vi "CIE2T-Config.vi"(0 "AO Channels":i32[](array[numeric]), 1 "Attenuation (dB)":dbl[](array[numeric]), 5 "DP Freqs":T1, 7 "Sampling Rate (Hz)":dbl=100000.0, 9 "Duration (s)":dbl=0.1, 11 "error in (no error)":errorcluster, 12 "Ear":T2) -> (2 "dt (ms)":dbl, 3 "df (kHz)":dbl, 4 "coerced f1 (kHz)":dbl, 6 "coerced f2 (kHz)":dbl, 10 "Mic Avg":dbl[][](array[numeric]), 15 "error out":errorcluster)   [LabVIEW 2020]
uses:
  Utility VIs/Type Defs/Left-Right ring.ctl
  Cochlear Function Test Suite/LV Source/DPOAE VIs/Typedefs/DP-Freqs.ctl
  Misc VIs/Connection Manager/Type Defs/Input sources.ctl
  PXI DAQ VIs/DAQ Engine VIs/PXI Globals.vi
  PXI DAQ VIs/DAQ Engine VIs/AO Gain and Multiplier VIs/PXI Multipliers to AO Gains (1D).vi
  PXI DAQ VIs/TDT VIs/TDT-Signal Bank Action.ctl
  Utility VIs/Math VIs/dB to Linear (scalar).vi
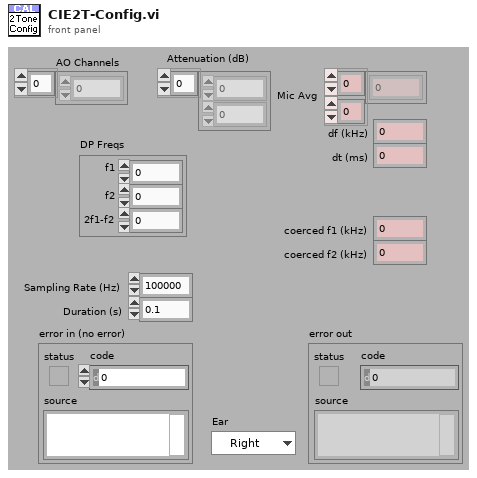
[diagram p1: front panel]
types:
  T1 = typedef "DP-Freqs.ctl" = cluster{"f1":dbl, "f2":dbl, "2f1-f2":dbl}
  T2 = typedef "Left-Right ring.ctl" = enum16{"Right", "Left"}
  T3 = typedef "Input sources.ctl" = u16
  T4 = typedef "TDT-Signal Bank Action.ctl" = enum16{"Init", "Write", "Read", "Rewrite", "Reset", "Recycle", "Ramp up", "Ramp down", "Zero"}
  T5 = typedef "TDT-Device Config.ctl" = cluster{"Output":T6, "Input":T8}
  T6 = typedef "TDT-Output source.ctl" = cluster{"Device":T7, "Num":i32}
  T7 = typedef "TDT-Device ID.ctl" = enum16{"None", "PA5", "RP2", "RL2", "RA16", "RV8", "RX5", "RX6", "RX7", "RX8", "RZ2", "RZ5", "RZ6"}
  T8 = typedef "TDT-Input source.ctl" = enum16{"Front Panel", "RA4LI", "RA16LI"}
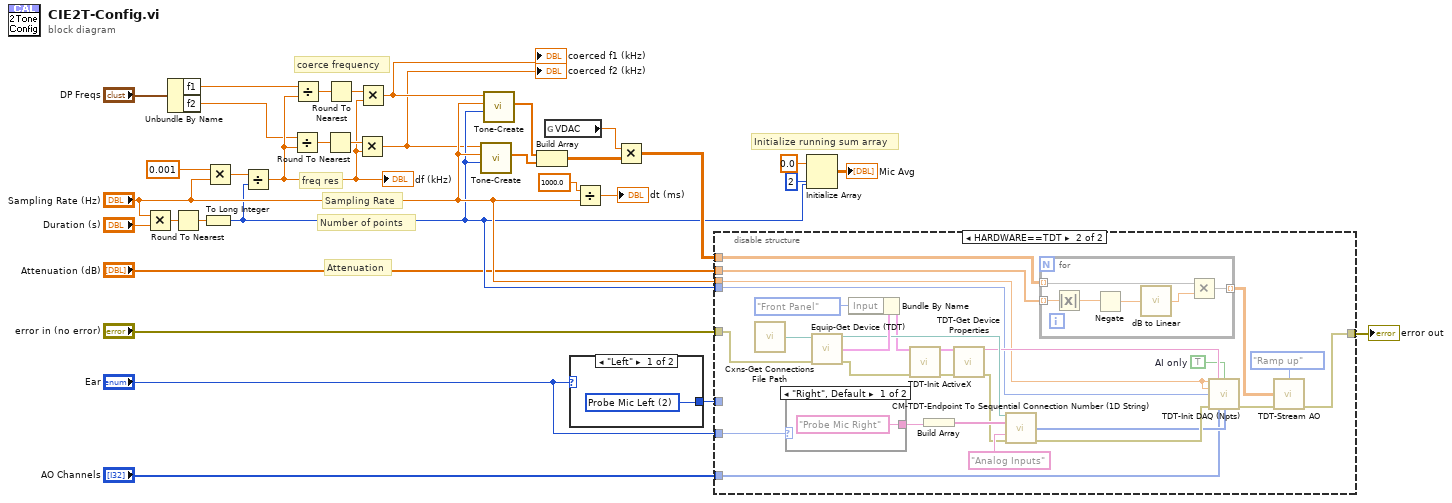
[diagram p0: block diagram]
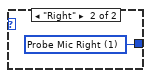
[diagram p2: hidden frame]
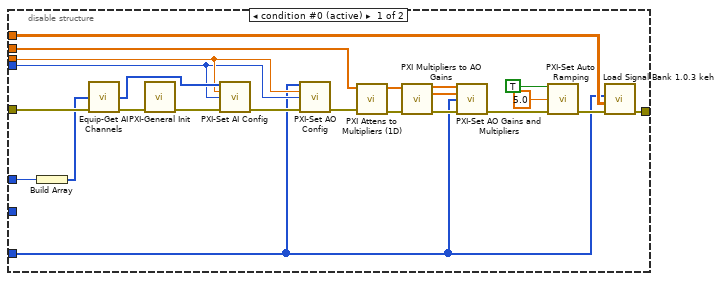
[diagram p3: hidden frame]
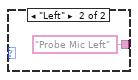
[diagram p4: hidden frame]
diagram:
  # "freq res"
  # "Attenuation"
  # "Sampling Rate"
  # "coerce frequency"
  # "Number of points"
  # "Initialize running sum array"
  n1 = Multiply(x="Sampling Rate (Hz)", y="Duration (s)") -> (x*y=w27:dbl)
  n2 = Unbundle By Name("DP Freqs") -> ("f1"=w6:dbl, "f2"=w5:dbl)
  n3 = Round To Nearest(number=w27) -> (nearest integer value=w26:dbl)
  n4 = To Long Integer(number=w26) -> (32bit integer=w11:i32)
  n5 = Multiply(x=0.001, y="Sampling Rate (Hz)") -> (x*y=w21:dbl)
  n6 = Divide(x=w21, y=w11) -> (x/y=w16:dbl)
  "df (kHz)" <- w16
  n7 = Divide(x=w5, y=w16) -> (x/y=w24:dbl)
  n8 = Divide(x=w6, y=w16) -> (x/y=w18:dbl)
  n9 = Round To Nearest(number=w24) -> (nearest integer value=w23:dbl)
  n10 = Round To Nearest(number=w18) -> (nearest integer value=w17:dbl)
  n11 = Multiply(x=w23, y=w16) -> (x*y=w8:dbl)
  "coerced f2 (kHz)" <- w8
  n12 = Multiply(x=w17, y=w16) -> (x*y=w9:dbl)
  "coerced f1 (kHz)" <- w9
  n13 = call "Tone-Create.vi"("Npts"=w11, "Sampling Rate (Hz)"="Sampling Rate (Hz)", "Frequency (kHz)"=w8) -> ("Waveform"=w22:dbl[])  [unwired: 7 in, 1 out]
  n14 = call "Tone-Create.vi"("Npts"=w11, "Sampling Rate (Hz)"="Sampling Rate (Hz)", "Frequency (kHz)"=w9) -> ("Waveform"=w15:dbl[])  [unwired: 7 in, 1 out]
  n15 = Build Array(w15, w22) -> (w10:dbl[][])
  n16 = global read "PXI Globals.vi" "VDAC"() -> (w13:dbl)
  n17 = case shown="\"Left\"" "Ear" {
    tunnel: [w34 w35] -> w2
    frame "Left" {
      w34 = T3 2 items=["--unused--", "Probe Mic Right", "Probe Mic Left", "Cal Mic", "ABR", "CAP Right", "CAP Left", "Startle piezo", "Temperature", "Heart rate"] ("Ring")
    }
    frame "Right" {
      w35 = T3 1 items=["--unused--", "Probe Mic Right", "Probe Mic Left", "Cal Mic", "ABR", "CAP Right", "CAP Left", "Startle piezo", "Temperature", "Heart rate"] ("Ring")
    }
  }
  n18 = Divide(x=1000.0, y="Sampling Rate (Hz)") -> (x/y=→"dt (ms)":dbl)
  n19 = Multiply(x=w13, y=w10) -> (x*y=w19:dbl[][])
  n20 = disable-structure shown="HARDWARE==TDT" {
    disable-tunnel: [w56 w68] -> w28
    disable-tunnel: w19 -> [w55 w66]
    disable-tunnel: "error in (no error)" -> [w54 w82]
    disable-tunnel: "Sampling Rate (Hz)" -> [w49 w74]
    disable-tunnel: w11 -> [w48 w73]
    disable-tunnel: "AO Channels" -> [w39 w70]
    disable-tunnel: "Attenuation (dB)" -> [w37 w67]
    disable-tunnel: w2 -> [w36 _]
    disable-tunnel: "Ear" -> [_ w64]
    frame condition #0 (active) {
      n21 = Build Array(w36) -> (w53:T3[])
      n22 = call "Equip-Get AI Channels.vi"("Inputs"=w53, "error in (no error)"=w54) -> ("AI Channels"=w51:i32[], "error out"=w38:errorcluster)  [unwired: 12 in]
      n23 = call "PXI-General Init.vi"("error in (no error)"=w38) -> ("error out"=w52:errorcluster)  [unwired: 10 in]
      n24 = call "PXI-Set AI Config.vi"("AI Channels"=w51, "Sampling Rate (Hz)"=w49, "Buffer Size"=w48, "error in (no error)"=w52) -> ("error out"=w50:errorcluster)  [unwired: 11 in]
      n25 = call "PXI-Set AO Config.vi"("AO Channels"=w39, "Sampling Rate (Hz)"=w49, "Buffer Size"=w48, "error in (no error)"=w50) -> ("error out"=w47:errorcluster)  [unwired: 11 in]
      n26 = call "PXI Attens to Multipliers (1D).vi"("error in (no error)"=w47, "Array of Attens"=w37) -> ("error out"=w58:errorcluster, "Multiplier setting"=w57:dbl[])  [unwired: 8 in]
      n27 = call-poly "PXI Multipliers to AO Gains.vi"("Multipliers in"=w57, "error in (no error)"=w58) -> ("Multipliers out"=w45:dbl[], "Gains"=w43:dbl[], "error out"=w46:errorcluster)  [unwired: 11 in]
      n28 = call "PXI-Set AO Gains and Multipliers.vi"("Multipliers"=w45, "Gains"=w43, "AO Channels"=w39, "error in (no error)"=w46) -> ("error out"=w44:errorcluster)  [unwired: 11 in]
      n29 = call "PXI-Set Auto Ramping.vi"("Auto ramp?"=TRUE, "Ramp duration (ms)"=5.0, "error in (no error)"=w44) -> ("error out"=w42:errorcluster)  [unwired: 12 in]
      n30 = call "Load Signal Bank 1.0.3 keh.vi"("error in (no error)"=w42, "Input array"=w55, "Active AO Array"=w39) -> ("error out"=w56:errorcluster)  [unwired: 6 in, 2 out]
    }
    frame condition #1 {
      w75 = TRUE  # AI only
      n31 = call "Cxns-Get Connections File Path.vi"() -> ("Path Out"=w83:path)  [unwired: 1 in]
      n32 = case shown="\"Right\", Default" w64 {
        tunnel: ["Probe Mic Right" "Probe Mic Left"] -> w63
        frame "Right", Default {
        }
        frame "Left" {
        }
      }
      n33 = call "Equip-Get Device (TDT).vi"("Path In"=w83, "error in (no error)"=w82) -> ("Path Out"=w79:path, "TDT-Device Config"=w81:T5, "error out"=w60:errorcluster)  [unwired: 11 in]
      n34 = Bundle By Name(cluster=w81, "Input"=enum16{"Front Panel", "RA4LI", "RA16LI"}."Front Panel") -> (w62:T5)
      n35 = call "TDT-Init ActiveX.vi"("TDT-Device Config"=w62, "error in (no error)"=w60) -> ("TDT-Device Config out"=w61:T5, "error out"=w59:errorcluster)  [unwired: 10 in, 2 out]
      n36 = Build Array(w63) -> (w80:string[])
      n37 = call "TDT-Get Device Properties.vi"("TDT-Device Config"=w61, "error in (no error)"=w59) -> ("Circuit File"=w76:string, "error out"=w78:errorcluster)  [unwired: 8 in, 4 out]
      n38 = call "CM-TDT-Endpoint To Sequential Connection Number (1D String).vi"("Path In"=w79, "Endpoints"=w80, "Section"="Analog Inputs", "error in (no error)"=w78) -> ("SeqCxnNum"=w71:i32[], "error out"=w72:errorcluster)  [unwired: 9 in, 1 out]
      n39 = for {
        tunnel: w67 -> [w89] mode=indexing
        tunnel: w66 -> [w93] mode=indexing
        tunnel: [w92] -> w65 mode=indexing
        n40 = Absolute Value(x=w89) -> (abs(x)=w90:dbl)
        n41 = Negate(x=w90) -> (-x=w91:dbl)
        n42 = call-poly "dB to Linear.vi"("dB"=w91) -> ("linear"=w88:dbl)
        n43 = Multiply(x=w93, y=w88) -> (x*y=w92:dbl[])
      }
      n44 = call "TDT-Init DAQ (Npts).vi"("AO Fs (Hz)"=w74, "Circuit"=w76, "AI only"=w75, "AI Fs (Hz)"=w74, "Num AO Pts"=w73, "error in (no error)"=w72, "AO Channels"=w70, "AI Channels"=w71) -> ("error out"=w69:errorcluster)  [unwired: 3 in, 4 out]
      n45 = call "TDT-Stream AO.vi"("Action"=TDT-Signal_Bank_Action."Ramp up", "Output array"=w65, "error in (no error)"=w69) -> ("error out"=w68:errorcluster)  [unwired: 12 in]
    }
  }
  "error out" <- w28
  n46 = Initialize Array(0.0 ("element"), 2 ("dimension size"), w11) -> (→"Mic Avg":dbl[][])
